vi "moveToInitialPos.vi"(8 "error in (no error)":errorcluster) -> (0 "error out":errorcluster)   [LabVIEW 2021]
doc: "André Romero - 2023\nandretec@ifsc.usp.br\nIFSC - USP"
uses:
  Global Motors.vi
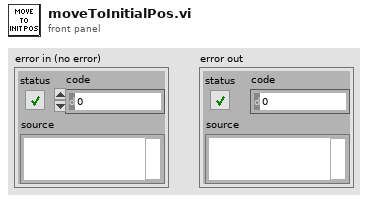
[diagram p1: front panel]
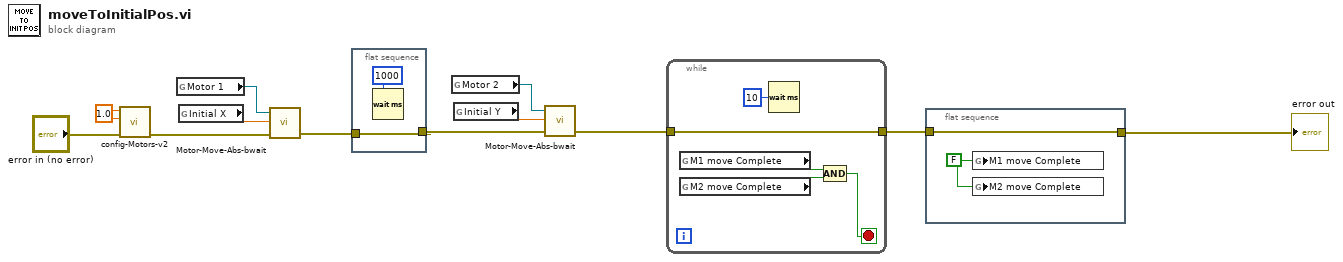
[diagram p0: block diagram]
diagram:
  w9 = sgl 1.0 ("Velocity")
  n1 = call "config-Motors-v2.vi"("error in"="error in (no error)", "Acc"=w9, "Velocity"=w9) -> ("error out"=w8:errorcluster)  [unwired: 8 in]
  n2 = global read "Global Motors.vi" "Motor 1"() -> (w1:refnum<k7>)
  n3 = global read "Global Motors.vi" "Initial X"() -> (w2:dbl)
  n4 = call "Motor-Move-Abs-bwait.vi"("error"=w8, "Posição"=w2, "MG17Motor A"=w1) -> ("error out"=w10:errorcluster)  [unwired: 1 in, 1 out]
  n5 = flat-sequence {
    tunnel: w10 -> [w14]
    tunnel: [w14] -> w11
    frame #0 {
      n6 = Wait (ms)(milliseconds to wait=u32 1000) -> ()  [unwired: 1 out]
    }
  }
  n7 = global read "Global Motors.vi" "Motor 2"() -> (w3:refnum<k7>)
  n8 = global read "Global Motors.vi" "Initial Y"() -> (w4:dbl)
  n9 = call "Motor-Move-Abs-bwait.vi"("error"=w11, "Posição"=w4, "MG17Motor A"=w3) -> ("error out"=w5:errorcluster)  [unwired: 1 in, 1 out]
  n10 = while {
    tunnel: w5 -> [w19]
    tunnel: [w19] -> w6
    stop <- w16 stop-if-true
    n11 = global read "Global Motors.vi" "M1 move Complete"() -> (w18:bool)
    n12 = global read "Global Motors.vi" "M2 move Complete"() -> (w17:bool)
    n13 = Wait (ms)(milliseconds to wait=u32 10) -> ()  [unwired: 1 out]
    n14 = Compound Arithmetic op=AND(w18, w17) -> (w16:bool)
  }
  n15 = flat-sequence {
    tunnel: w6 -> [w20]
    tunnel: [w20] -> w12
    frame #0 {
      w21 = FALSE ("M1 move Complete")
      n16 = global write "Global Motors.vi" "M1 move Complete"(w21) -> ()
      n17 = global write "Global Motors.vi" "M2 move Complete"(w21) -> ()
    }
  }
  "error out" <- w12
